vi "html_write.vi"() -> ()   [LabVIEW 2017]
uses:
  <vilib>/httpClient/LabVIEWHTTPClient.lvlib
panel:
  out "error out":errorcluster
  out "headers":string
  out "body":string
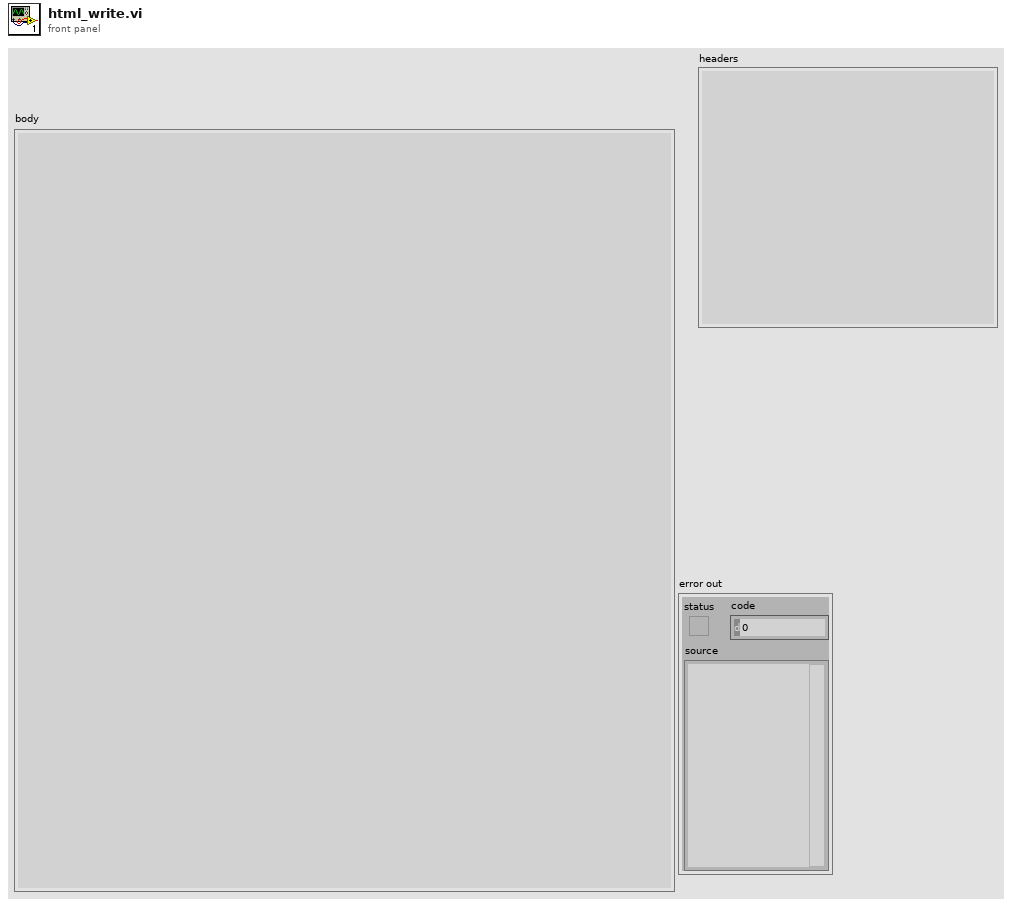
[diagram p1: front panel]
types:
  T1 = cluster{"Name":string, "Value":string, "File":path, "Filename":string, "MIME type":string}
  T2 = cluster{"Name":string, "Value":string, "File":path, "Filename":string, "MIME type":string}[]
  T3 = typedef "LabVIEWHTTPClient.lvlib/ClientHandle.ctl" = refnum<k1>
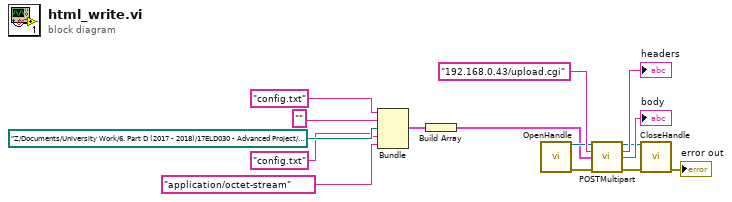
[diagram p0: block diagram]
diagram:
  n1 = Bundle("Name"="config.txt", "Value"="", "File"=path "Z:/Documents/University Work/6. Part D (2017 - 2018)/17ELD030 - Advanced Project/LabVIEW/config.txt", "Filename"="config.txt", "MIME type"="application/octet-stream") -> (w1:T1)  [unwired: 1 in]
  n2 = Build Array(w1) -> (w7:T2)
  n3 = call <vilib>:"OpenHandle.vi"() -> ("client handle out"=w14:T3, "error out"=w11:errorcluster)  [unwired: 14 in]
  n4 = call <vilib>:"POSTMultipart.vi"("client handle"=w14, "url"="192.168.0.43/upload.cgi", "data"=w7, "error in (no error)"=w11) -> ("client handle out"=w10:T3, "headers"=→"headers":string, "body"=→"body":string, "error out"=w9:errorcluster)  [unwired: 8 in]
  n5 = call <vilib>:"CloseHandle.vi"("client handle"=w10, "error in (no error)"=w9) -> ("error out"=→"error out":errorcluster)  [unwired: 13 in]
